vi "test_libssh2_channel_forward_cancel.vi"() -> ()   [LabVIEW 2013, in "libssh2_integration_tests.lvlib"]
uses:
  libssh2_integration_tests.lvlib
  <vilib>/addons/_JKI Toolkits/Caraya/classes/Test/Test.lvclass
  support/support.lvlib
  <vilib>/addons/_JKI Toolkits/Caraya/classes/Assert/Assert.lvclass
  libssh2/libssh2.lvlib
panel:
  out "error out":errorcluster
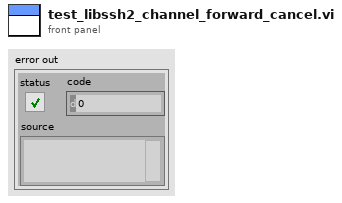
[diagram p1: front panel]
types:
  T1 = typedef "libssh2.lvlib/Session Refnum.ctl" = refnum<k1>
  T2 = typedef "libssh2.lvlib/Listener Refnum.ctl" = refnum<k1>
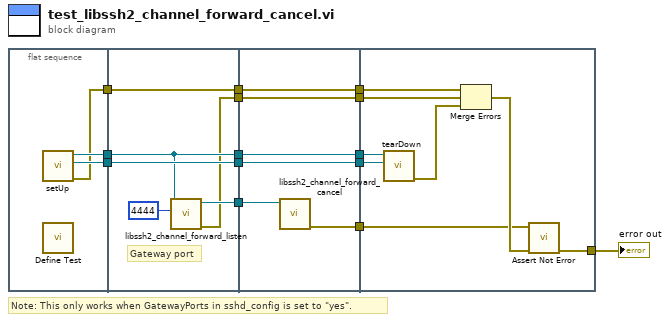
[diagram p0: block diagram]
diagram:
  # "Note: This only works when GatewayPorts in sshd_config is set to \"yes\"."
  n1 = flat-sequence {
    tunnel: [w17] -> w14
    tunnel: [w16] -> w13
    tunnel: [w15] -> w12
    tunnel: w14 -> [w21]
    tunnel: w13 -> [w23]
    tunnel: [w21] -> w5
    tunnel: [w23] -> w4
    tunnel: w12 -> [w22]
    tunnel: [w22] -> w3
    tunnel: [w19] -> w2
    tunnel: [w20] -> w1
    tunnel: w5 -> [w29]
    tunnel: [w29] -> w10
    tunnel: w4 -> [w28]
    tunnel: [w28] -> w9
    tunnel: w3 -> [w27]
    tunnel: [w27] -> w8
    tunnel: w2 -> [w26]
    tunnel: [w26] -> w7
    tunnel: w1 -> [w25]
    tunnel: [w24] -> w6
    tunnel: w10 -> [w37]
    tunnel: w9 -> [w36]
    tunnel: [w35] -> w11
    tunnel: w8 -> [w33]
    tunnel: w7 -> [w31]
    tunnel: w6 -> [w30]
    frame #0 {
      n2 = call "setUp.vi"() -> ("error out"=w15:errorcluster, "connection ID"=w16:refnum<k5>, "session"=w17:T1)  [unwired: 9 in]
      n3 = call <vilib>:"Define Test.vi"() -> ()  [unwired: 10 in, 2 out]
    }
    frame #1 {
      # "Gateway port"
      n4 = call "libssh2_channel_forward_listen.vi"("port in"=4444, "session"=w21) -> ("error out"=w19:errorcluster, "listener"=w20:T2)  [unwired: 7 in, 1 out]
    }
    frame #2 {
      n5 = call "libssh2_channel_forward_cancel.vi"("listener"=w25) -> ("error out"=w24:errorcluster)  [unwired: 10 in]
    }
    frame #3 {
      n6 = call "tearDown.vi"("connection ID"=w36, "session"=w37) -> ("error out"=w34:errorcluster)  [unwired: 9 in]
      n7 = Merge Errors(w33, w31, w34) -> (w32:errorcluster)
      n8 = call <vilib>:"Assert Not Error.vi"("error in (no error)"=w32, "Not Error?"=w30) -> ("error out"=w35:errorcluster)  [unwired: 8 in, 1 out]
    }
  }
  "error out" <- w11
